vi "MPUSBGetDeviceCount.vi"(8 "error in (no error)":errorcluster, 11 "pVID_PID":string="vid_04d8&pid_fc5f") -> (0 "error out":errorcluster, 3 "return_value":u32)   [LabVIEW 2019]
doc: "Returns count of devices found\n\nWritten by: Complete Automated Solutions\nwww.CompleteAutomatedSolutions.com"
uses:
  mpusbapi.dll
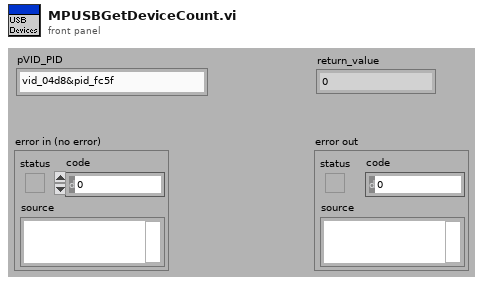
[diagram p1: front panel]
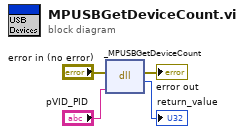
[diagram p0: block diagram]
diagram:
  n1 = dll-call lib="C:/Users/z003r4zd/Desktop/Point Contact Mods 2019/Automation/Actuonix/LAC+Labview+Example/Actuonix_LAC_LabVIEW_Example/USB_VIs/mpusbapi.dll" fn="_MPUSBGetDeviceCount"(error in="error in (no error)", "pVID_PID"="pVID_PID") -> (error out=→"error out":errorcluster, "return_value"=→"return_value":u32)  [unwired: 3 in, 1 out]
